vi "Protocol.Read Queued Processed Outgoing Messages.vi"(8 "error in (no error)":errorcluster, 10 "timeout in ms (-1)":i32, 11 "J1939 Cluster":T2) -> (0 "error out":errorcluster, 2 "timed out?":bool, 3 "Frame":T1 {"Identifier" format="%08x"})   [LabVIEW 2019, in "J1939 Addon Engine.lvlib"]
uses:
  J1939 Addon Engine.lvlib
  Types/Protocol.Refs.ctl
  Support Libraries/J1939 Utilities/Types/CAN Outgoing Message Cluster.ctl
  Types/Protocol.RQST Lookup Table Reference.ctl
  Types/Protocol.Address Table Reference.ctl
  Support Libraries/J1939 Utilities/J1939 Utilities.lvlib
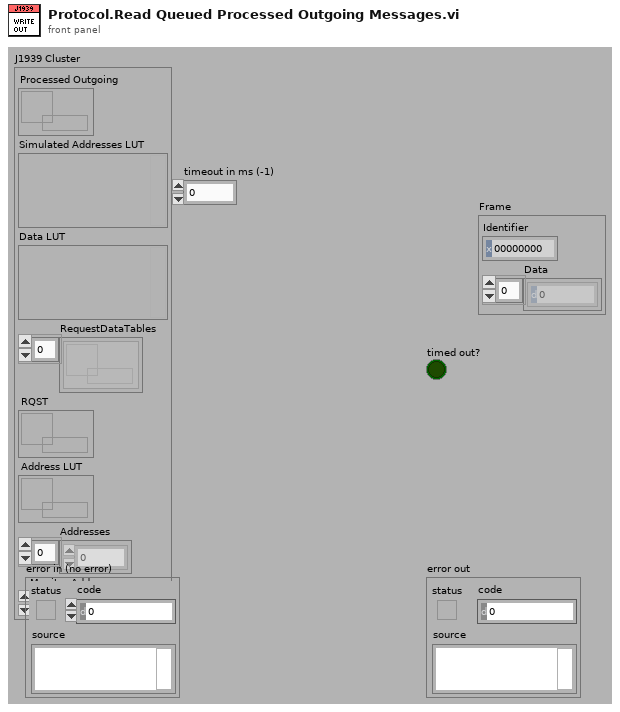
[diagram p1: front panel]
types:
  T1 = typedef "J1939 Utilities.lvlib/CAN Outgoing Message Cluster.ctl" = cluster{"Identifier":u32, "Data":u8[]}
  T2 = typedef "J1939 Addon Engine.lvlib/Protocol.Refs.ctl" = cluster{"Processed Outgoing":refnum<queue>, "Simulated Addresses LUT":variant, "Data LUT":variant, "RequestDataTables":refnum<k33>[], "RQST":T3, "Address LUT":T4, "Addresses":u8[], "Monitor Address":u8}
  T3 = typedef "J1939 Addon Engine.lvlib/Protocol.RQST Lookup Table Reference.ctl" = refnum<data-value>
  T4 = typedef "J1939 Addon Engine.lvlib/Protocol.Address Table Reference.ctl" = refnum<data-value>
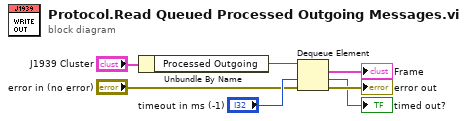
[diagram p0: block diagram]
diagram:
  n1 = Unbundle By Name("J1939 Cluster") -> ("Processed Outgoing"=w1:refnum<queue>)
  n2 = Dequeue Element(queue=w1, timeout in ms (-1)="timeout in ms (-1)", error in (no error)="error in (no error)") -> (element=→"Frame":T1, timed out?=→"timed out?":bool, error out=→"error out":errorcluster)  [unwired: 1 out]
